vi "UDP to Rx.vi"(7 "Data Conversion":T1, 8 "error in (no error)":errorcluster, 10 "Rx String":string) -> (0 "error out":errorcluster, 2 "Rx Array":dbl[](array[numeric]), 5 "Data Conversion out":T1)   [LabVIEW 2016, in "UDP-Custom-Device Engine.lvlib"]
uses:
  UDP-Custom-Device Engine.lvlib
  Types/Engine - Data Conversion Config.ctl
  <vilib>/NI Veristand/VeriStand Data/Library/Byte Buffer/Byte Buffer.lvclass
  <vilib>/NI Veristand/VeriStand Data/Library/Byte Buffer/Byte Buffer.Mapping.ctl
  <vilib>/NI Veristand/VeriStand Data/Library/Typedefs/Typedefs.Data Types.ctl
  <vilib>/NI Veristand/VeriStand Data/Library/Byte Buffer/Byte Buffer.lvclass/Byte Buffer.ctl
  <vilib>/NI Veristand/VeriStand Data/Library/Pointer Operations/Pointer.Read (DBL).vi
  <vilib>/NI Veristand/VeriStand Data/Library/Byte Buffer/Byte Buffer.Read.Typed Array.vi
  <vilib>/NI Veristand/VeriStand Data/Library/Memory Management/Memory Management.MoveDblBlock.Read (Double).vi
  <vilib>/NI Veristand/VeriStand Data/Library/Utilities/Utilities.Buffer.Double.vi
  <vilib>/NI Veristand/VeriStand Data/Library/Pointer Operations/Pointer.In-Place Read (DBL).vi
  <vilib>/NI Veristand/VeriStand Data/Library/Utilities/Utilities.Sizeof.Array.vi
  <vilib>/NI Veristand/VeriStand Data/Library/Byte Buffer/Byte Buffer.Read.vi
  <vilib>/NI Veristand/VeriStand Data/Library/Byte Buffer/Byte Buffer.Read (1D Boolean).vi
  <vilib>/NI Veristand/VeriStand Data/Library/Type Conversion/Type Conversion.To Double.Subset.vi
  <vilib>/NI Veristand/VeriStand Data/Library/Type Conversion/Type Conversion.To Double.Subset (1D Boolean).vi
  <vilib>/NI Veristand/VeriStand Data/Library/Byte Buffer/Byte Buffer.Read (1D SGL).vi
  <vilib>/NI Veristand/VeriStand Data/Library/Type Conversion/Type Conversion.To Double.Subset (1D SGL).vi
  <vilib>/NI Veristand/VeriStand Data/Library/Byte Buffer/Byte Buffer.Read (1D DBL).vi
  <vilib>/NI Veristand/VeriStand Data/Library/Byte Buffer/Byte Buffer.Read (1D I8).vi
  <vilib>/NI Veristand/VeriStand Data/Library/Type Conversion/Type Conversion.To Double.Subset (1D I8).vi
  <vilib>/NI Veristand/VeriStand Data/Library/Byte Buffer/Byte Buffer.Read (1D I16).vi
  <vilib>/NI Veristand/VeriStand Data/Library/Type Conversion/Type Conversion.To Double.Subset (1D I16).vi
  <vilib>/NI Veristand/VeriStand Data/Library/Byte Buffer/Byte Buffer.Read (1D I32).vi
  <vilib>/NI Veristand/VeriStand Data/Library/Type Conversion/Type Conversion.To Double.Subset (1D I32).vi
  <vilib>/NI Veristand/VeriStand Data/Library/Byte Buffer/Byte Buffer.Read (1D I64).vi
  <vilib>/NI Veristand/VeriStand Data/Library/Type Conversion/Type Conversion.To Double.Subset (1D I64).vi
  <vilib>/NI Veristand/VeriStand Data/Library/Byte Buffer/Byte Buffer.Read (1D U8).vi
  <vilib>/NI Veristand/VeriStand Data/Library/Type Conversion/Type Conversion.To Double.Subset (1D U8).vi
  <vilib>/NI Veristand/VeriStand Data/Library/Byte Buffer/Byte Buffer.Read (1D U16).vi
  <vilib>/NI Veristand/VeriStand Data/Library/Type Conversion/Type Conversion.To Double.Subset (1D U16).vi
  <vilib>/NI Veristand/VeriStand Data/Library/Byte Buffer/Byte Buffer.Read (1D U32).vi
  <vilib>/NI Veristand/VeriStand Data/Library/Type Conversion/Type Conversion.To Double.Subset (1D U32).vi
  <vilib>/NI Veristand/VeriStand Data/Library/Byte Buffer/Byte Buffer.Read (1D U64).vi
  <vilib>/NI Veristand/VeriStand Data/Library/Type Conversion/Type Conversion.To Double.Subset (1D U64).vi
  <vilib>/NI Veristand/VeriStand Data/Library/Utilities/Utilities.Sizeof.Scalar.vi
  <vilib>/NI Veristand/VeriStand Data/Library/Type Conversion/Type Conversion.To Double.vi
  <vilib>/NI Veristand/VeriStand Data/Library/Type Conversion/Type Conversion.To Double (1D Boolean).vi
  <vilib>/NI Veristand/VeriStand Data/Library/Type Conversion/Type Conversion.To Double (1D SGL).vi
  <vilib>/NI Veristand/VeriStand Data/Library/Type Conversion/Type Conversion.To Double (1D I8).vi
  <vilib>/NI Veristand/VeriStand Data/Library/Type Conversion/Type Conversion.To Double (1D I16).vi
  <vilib>/NI Veristand/VeriStand Data/Library/Type Conversion/Type Conversion.To Double (1D I32).vi
  <vilib>/NI Veristand/VeriStand Data/Library/Type Conversion/Type Conversion.To Double (1D I64).vi
  <vilib>/NI Veristand/VeriStand Data/Library/Type Conversion/Type Conversion.To Double (1D U8).vi
  <vilib>/NI Veristand/VeriStand Data/Library/Type Conversion/Type Conversion.To Double (1D U16).vi
  <vilib>/NI Veristand/VeriStand Data/Library/Type Conversion/Type Conversion.To Double (1D U32).vi
  <vilib>/NI Veristand/VeriStand Data/Library/Type Conversion/Type Conversion.To Double (1D U64).vi
  <vilib>/NI Veristand/VeriStand Data/Library/Memory Management/Memory Management.Handle Return.vi
  <vilib>/NI Veristand/VeriStand Data/Library/VeriStand Data.lvlib
panel:
  out "Diagnostics":dbl[](array[numeric])
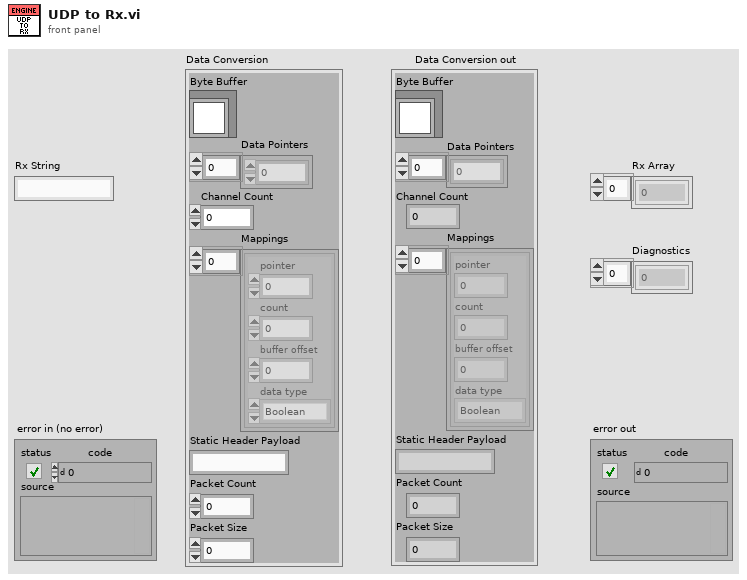
[diagram p1: front panel]
types:
  T1 = typedef "UDP-Custom-Device Engine.lvlib/Engine - Data Conversion Config.ctl" = cluster{"Byte Buffer":refnum<class "Byte Buffer.lvclass">, "Data Pointers":u64[], "Channel Count":i32, "Mappings":T2[], "Static Header Payload":string, "Packet Count":dbl, "Packet Size":i32}
  T2 = typedef "VeriStand Data.lvlib/Byte Buffer.lvclass/Byte Buffer.Mapping.ctl" = cluster{"pointer":u64, "count":i32, "buffer offset":i32, "data type":T3}
  T3 = typedef "VeriStand Data.lvlib/Typedefs.Data Types.ctl" = enum16{"Boolean", "Single", "Double", "I8", "I16", "I32", "I64", "U8", "U16", "U32", "U64"}
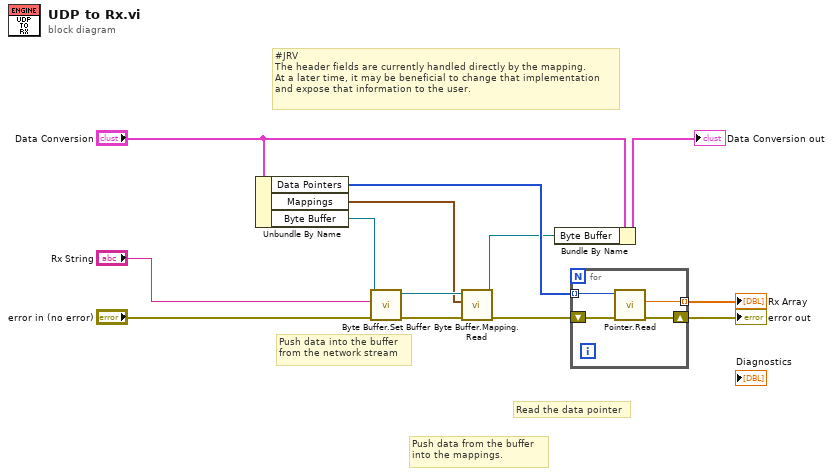
[diagram p0: block diagram]
diagram:
  # "#JRV\nThe header fields are currently handled directly by the mapping.\nAt a later time, it may be beneficial to change that implementation\nand expose that information to the user."
  # "Read the data pointer"
  # "Push data from the buffer\ninto the mappings."
  # "Push data into the buffer\nfrom the network stream"
  n1 = Unbundle By Name("Data Conversion") -> ("Data Pointers"=w2:u64[], "Mappings"=w5:T2[], "Byte Buffer"=w7:refnum<class "Byte Buffer.lvclass">)
  n2 = call <vilib>:"Byte Buffer.Set Buffer.vi"("error in (no error)"="error in (no error)", "buffer"="Rx String", "Byte Buffer in"=w7) -> ("error out"=w4:errorcluster, "Byte Buffer out"=w6:refnum<class "Byte Buffer.lvclass">)  [unwired: 7 in]
  n3 = call <vilib>:"Byte Buffer.Mapping.Read.vi"("error in (no error)"=w4, "mappings"=w5, "Byte Buffer in"=w6) -> ("error out"=w3:errorcluster, "Byte Buffer out"=w1:refnum<class "Byte Buffer.lvclass">)  [unwired: 6 in, 1 out]
  n4 = Bundle By Name(cluster="Data Conversion", "Byte Buffer"=w1) -> (→"Data Conversion out":T1)
  n5 = for {
    tunnel: [w16] -> w10 mode=indexing
    tunnel: w2 -> [w14] mode=indexing
    shift-right: [w17] -> w11
    shift-left: w3 -> [w15]
    n6 = call-poly <vilib>:"Pointer.Read.vi"("error in (no error)"=w15, "pointer in"=w14) -> ("error out"=w17:errorcluster, "value"=w16:dbl)  [unwired: 7 in, 1 out]
  }
  "error out" <- w11
  "Rx Array" <- w10
